vi "SetMultiVoltage_MultiVoltageSource.vi"(0 "VISA Refnum in":refnum<visa-resource-name>, 1 "Channel Value 6":dbl=0.2, 2 "Channel Value 7":dbl=0.2, 5 "Channel Value 5":dbl=0.2, 7 "Channel Value 4":dbl=0.2, 9 "Channel Value 3":dbl=0.2, 11 "error in (no error)":errorcluster, 12 "Channel Value 2":dbl=0.2, 13 "Channel Value":dbl=0.2) -> (4 "VISA Refnum out":refnum<visa-resource-name>, 15 "error out":errorcluster)   [LabVIEW 2020]
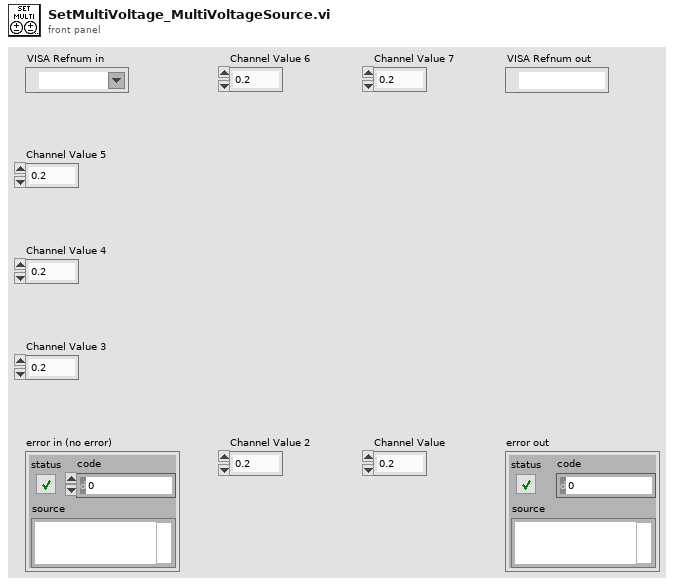
[diagram p1: front panel]
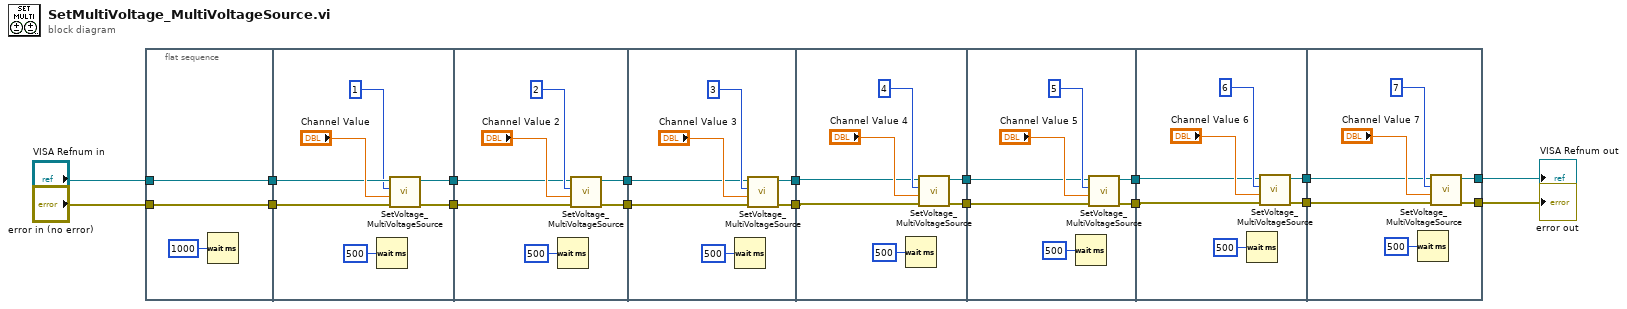
[diagram p0: block diagram]
diagram:
  n1 = flat-sequence {
    tunnel: "error in (no error)" -> [w20]
    tunnel: "VISA Refnum in" -> [w21]
    tunnel: [w21] -> w2
    tunnel: [w20] -> w1
    tunnel: [w25] -> w18
    tunnel: [w24] -> w17
    tunnel: w2 -> [w27]
    tunnel: w1 -> [w26]
    tunnel: w18 -> [w32]
    tunnel: w17 -> [w31]
    tunnel: [w30] -> w16
    tunnel: [w29] -> w15
    tunnel: w16 -> [w38]
    tunnel: w15 -> [w39]
    tunnel: [w37] -> w14
    tunnel: [w36] -> w13
    tunnel: w14 -> [w46]
    tunnel: w13 -> [w45]
    tunnel: [w44] -> w12
    tunnel: [w43] -> w11
    tunnel: w12 -> [w53]
    tunnel: w11 -> [w52]
    tunnel: [w51] -> w10
    tunnel: [w50] -> w9
    tunnel: w10 -> [w60]
    tunnel: w9 -> [w59]
    tunnel: [w58] -> w8
    tunnel: [w57] -> w7
    tunnel: w8 -> [w67]
    tunnel: w7 -> [w66]
    tunnel: [w65] -> w5
    tunnel: [w64] -> w6
    frame #0 {
      n2 = Wait (ms)(milliseconds to wait=u32 1000) -> ()  [unwired: 1 out]
    }
    frame #1 {
      n3 = Wait (ms)(milliseconds to wait=u32 500) -> ()  [unwired: 1 out]
      n4 = call "SetVoltage_MultiVoltageSource.vi"("error in (no error)"=w26, "Channel Value"="Channel Value", "Channel"=1, "VISA Refnum in"=w27) -> ("error out"=w24:errorcluster, "VISA Refnum out"=w25:refnum<visa-resource-name>)  [unwired: 6 in]
    }
    frame #2 {
      n5 = Wait (ms)(milliseconds to wait=u32 500) -> ()  [unwired: 1 out]
      n6 = call "SetVoltage_MultiVoltageSource.vi"("error in (no error)"=w31, "Channel Value"="Channel Value 2", "Channel"=2, "VISA Refnum in"=w32) -> ("error out"=w29:errorcluster, "VISA Refnum out"=w30:refnum<visa-resource-name>)  [unwired: 6 in]
    }
    frame #3 {
      n7 = Wait (ms)(milliseconds to wait=u32 500) -> ()  [unwired: 1 out]
      n8 = call "SetVoltage_MultiVoltageSource.vi"("error in (no error)"=w39, "Channel Value"="Channel Value 3", "Channel"=3, "VISA Refnum in"=w38) -> ("error out"=w36:errorcluster, "VISA Refnum out"=w37:refnum<visa-resource-name>)  [unwired: 6 in]
    }
    frame #4 {
      n9 = Wait (ms)(milliseconds to wait=u32 500) -> ()  [unwired: 1 out]
      n10 = call "SetVoltage_MultiVoltageSource.vi"("error in (no error)"=w45, "Channel Value"="Channel Value 4", "Channel"=4, "VISA Refnum in"=w46) -> ("error out"=w43:errorcluster, "VISA Refnum out"=w44:refnum<visa-resource-name>)  [unwired: 6 in]
    }
    frame #5 {
      n11 = Wait (ms)(milliseconds to wait=u32 500) -> ()  [unwired: 1 out]
      n12 = call "SetVoltage_MultiVoltageSource.vi"("error in (no error)"=w52, "Channel Value"="Channel Value 5", "Channel"=5, "VISA Refnum in"=w53) -> ("error out"=w50:errorcluster, "VISA Refnum out"=w51:refnum<visa-resource-name>)  [unwired: 6 in]
    }
    frame #6 {
      n13 = Wait (ms)(milliseconds to wait=u32 500) -> ()  [unwired: 1 out]
      n14 = call "SetVoltage_MultiVoltageSource.vi"("error in (no error)"=w59, "Channel Value"="Channel Value 6", "Channel"=6, "VISA Refnum in"=w60) -> ("error out"=w57:errorcluster, "VISA Refnum out"=w58:refnum<visa-resource-name>)  [unwired: 6 in]
    }
    frame #7 {
      n15 = Wait (ms)(milliseconds to wait=u32 500) -> ()  [unwired: 1 out]
      n16 = call "SetVoltage_MultiVoltageSource.vi"("error in (no error)"=w66, "Channel Value"="Channel Value 7", "Channel"=7, "VISA Refnum in"=w67) -> ("error out"=w64:errorcluster, "VISA Refnum out"=w65:refnum<visa-resource-name>)  [unwired: 6 in]
    }
  }
  "error out" <- w6
  "VISA Refnum out" <- w5
